vi "RockPaperScissors.vi"() -> ()   [LabVIEW 2021]
uses:
  <vilib>/numeric/Random Number (Range) DBL.vi
  <vilib>/Instr/_visa.llb/VISA Configure Serial Port (Instr).vi
panel:
  in  "Train":bool
  out "Output Selection 2":i32
  out "Output Selection 1":i32
  in  "Tab Control":enum32{"Play"}(tab)
  in  "Ready to Play":bool
  in  "User":picture
  in  "Computer":picture
  in  "Ring":u16(ring) items=["Scissors", "Paper", "Rock"]
  in  "Done":bool
  in  "VISA resource name":refnum<visa-resource-name>
  # "READY TO PLAY"
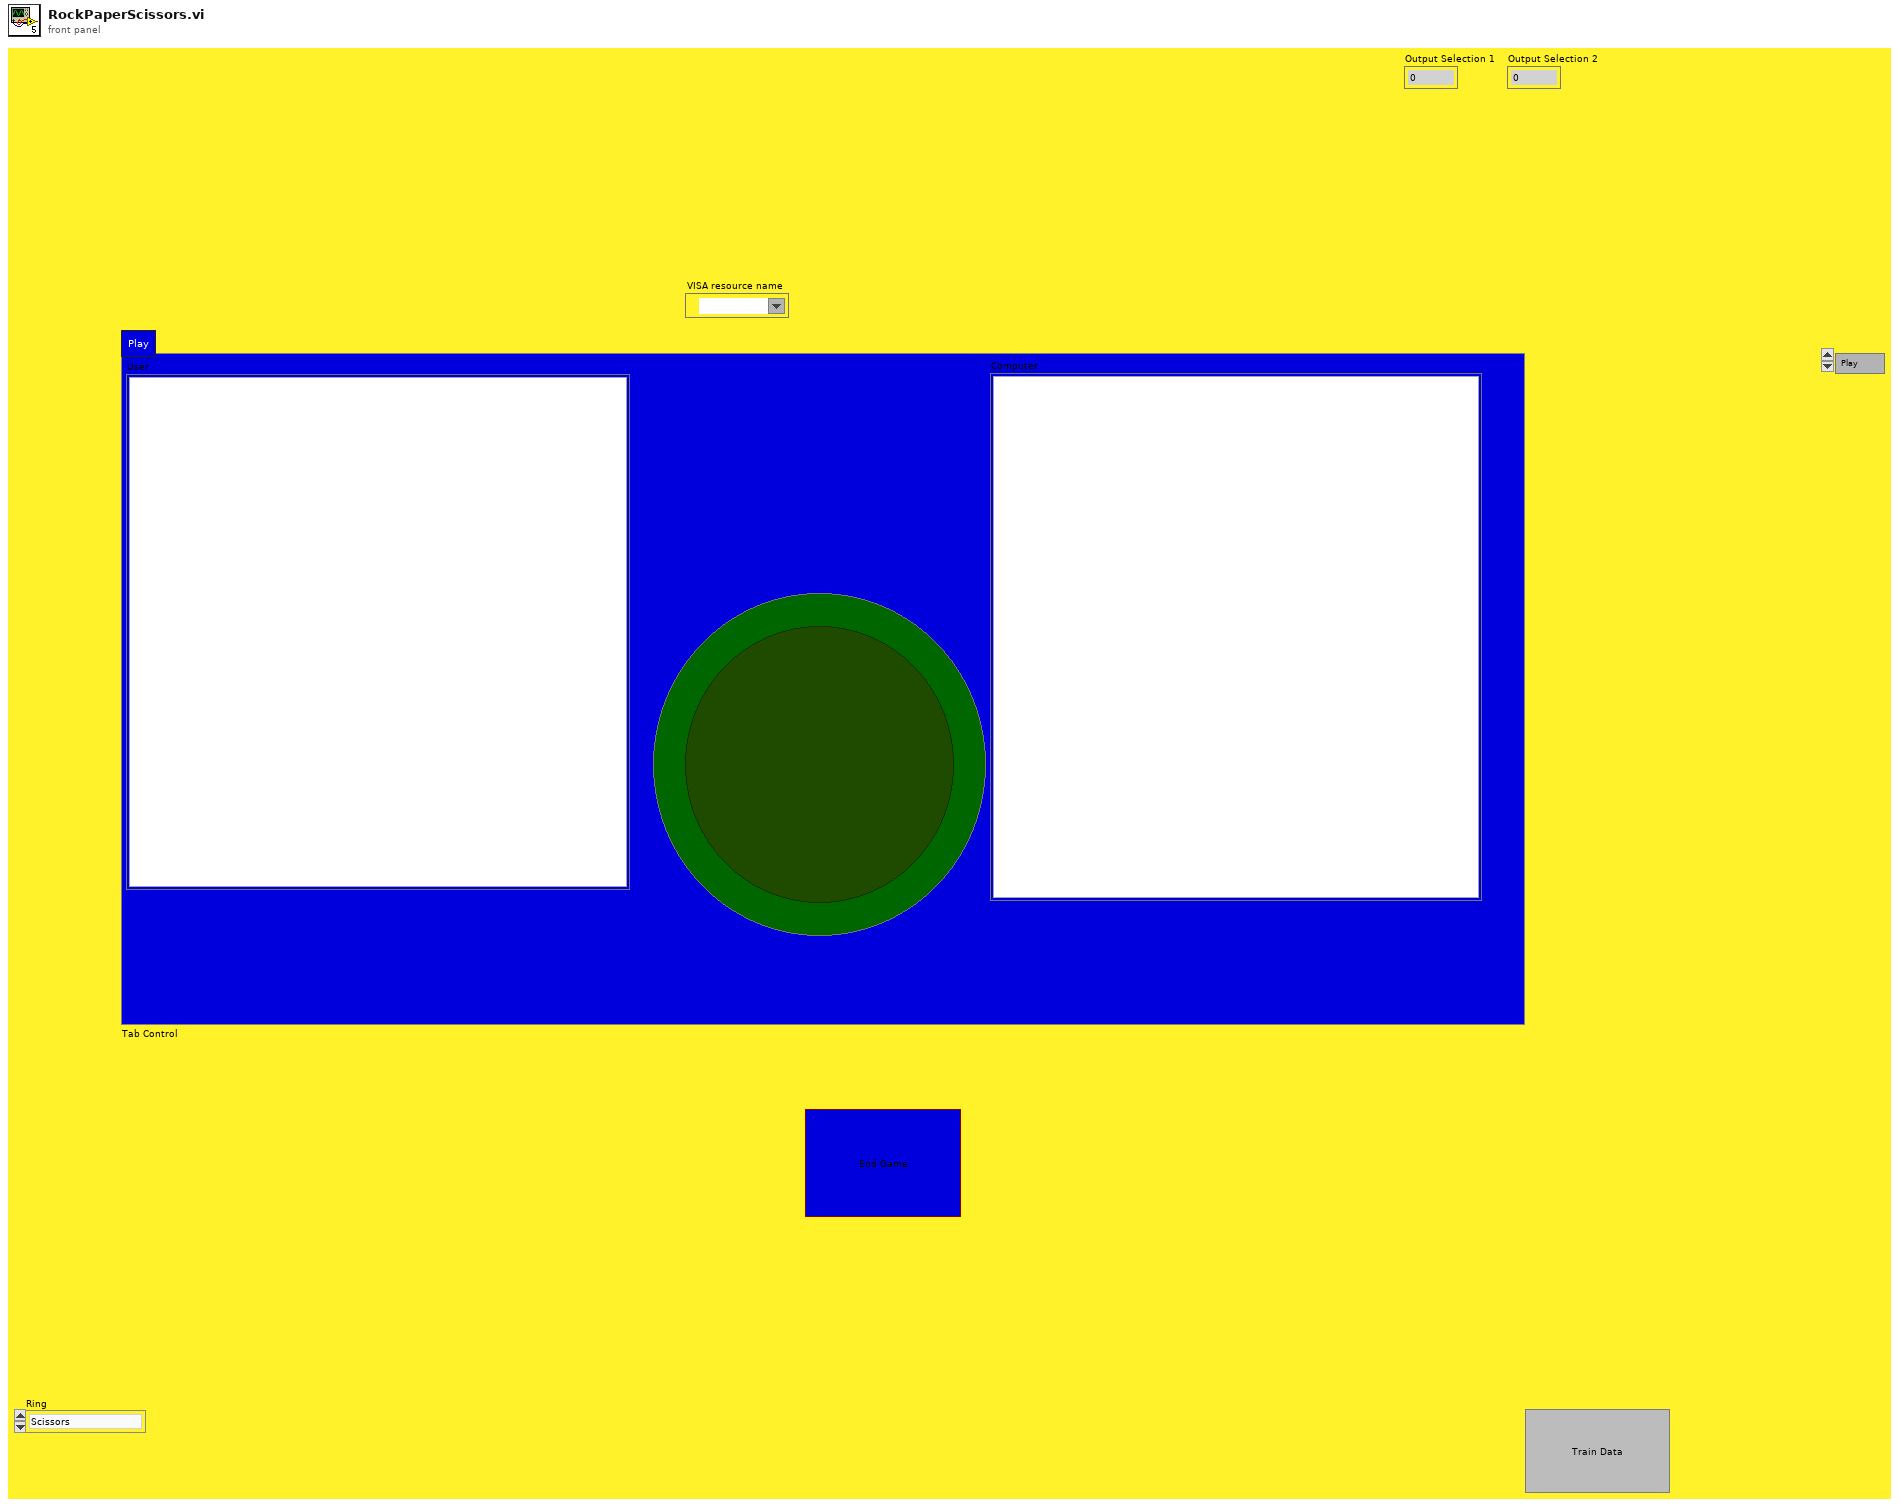
[diagram p1: front panel]
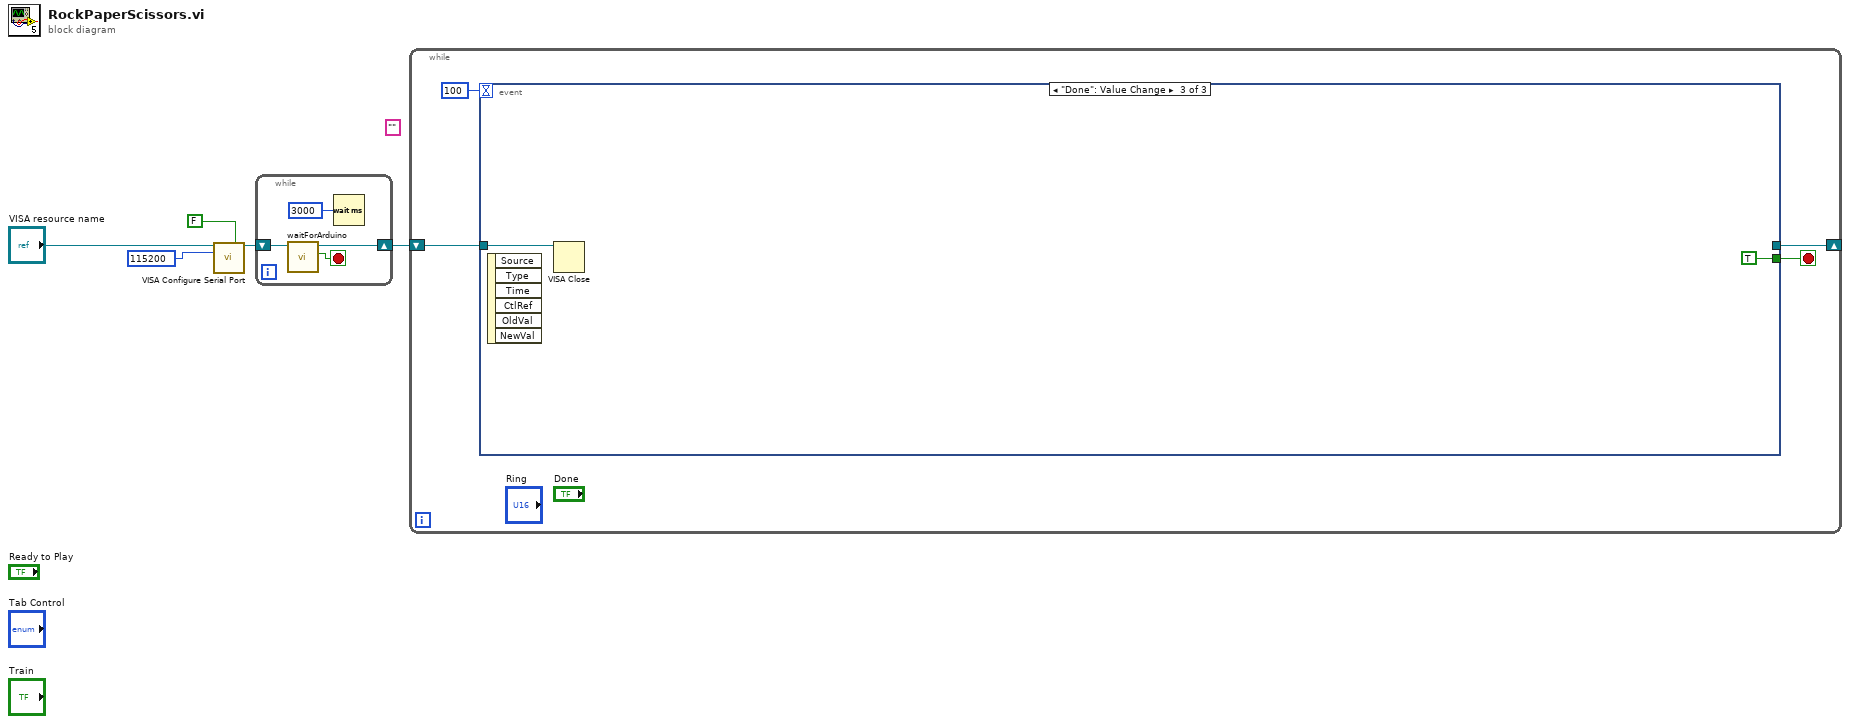
[diagram p0: block diagram]
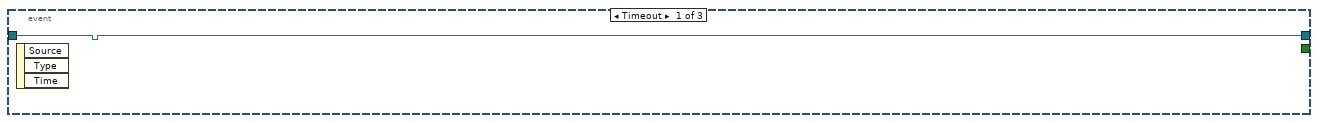
[diagram p2: hidden frame]
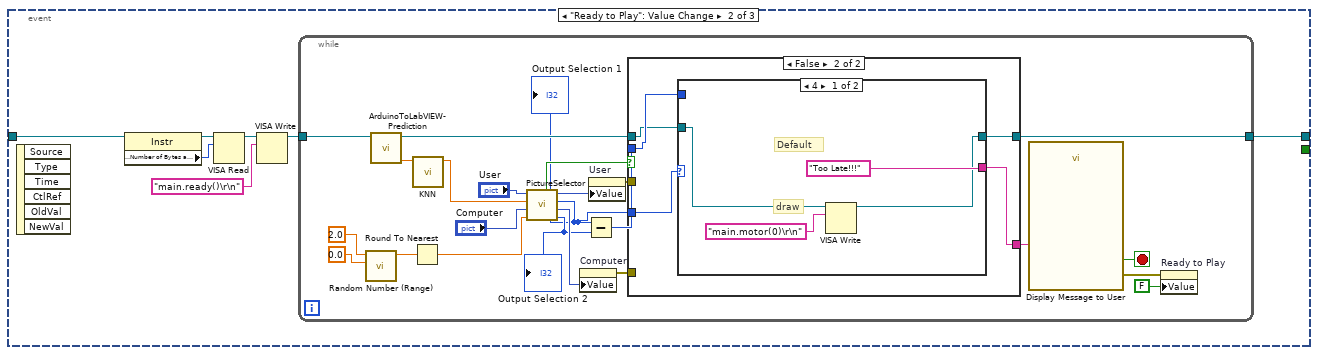
[diagram p3: hidden frame]
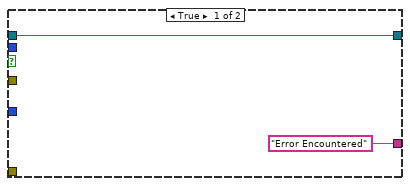
[diagram p4: hidden frame]
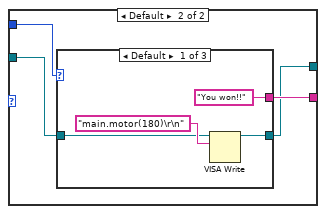
[diagram p5: hidden frame]
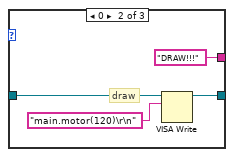
[diagram p6: hidden frame]
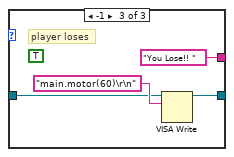
[diagram p7: hidden frame]
diagram:
  (unwired) ""
  n1 = call-poly "VISA Configure Serial Port"("VISA resource name"="VISA resource name", "Enable Termination\nChar (T)"=FALSE ("Enable Termination\nChar (T)"), "baud rate (9600)"=u32 115200) -> ("VISA resource name out"=w2:refnum<visa-resource-name>)  [unwired: 11 in, 1 out]
  n2 = while {
    shift-right: [w8] -> w1
    shift-left: w2 -> [w9]
    stop <- w7 stop-if-true
    n3 = call "waitForArduino.vi"("VISA Refnum in"=w9) -> ("Boolean"=w7:bool, "VISA Refnum out"=w8:refnum<visa-resource-name>)  [unwired: 9 in]
    n4 = Wait (ms)(milliseconds to wait=u32 3000) -> ()  [unwired: 1 out]
  }
  n5 = while {
    shift-right: [w11] -> _
    shift-left: w1 -> [w13]
    stop <- w12 stop-if-true
    n6 = event shown="[2] \"Done\": Value Change" {
      selector: _ -> [_ _ _]
      dyn-events: _ -> [_ _ _]
      timeout: 100 -> [_ _ _]
      tunnel: w13 -> [w14 w18 w72]
      tunnel: [_ _ TRUE] -> w12
      tunnel: [w14 w19 _] -> w11
      event Timeout {
        n7 = event-data() -> ()  [unwired: 1 in, 3 out]
      }
      event "Ready to Play": Value Change {
        n8 = event-data() -> ()  [unwired: 1 in, 6 out]
        n9 = property class="Instr"(reference=w18) -> (reference out=w17:refnum<visa-resource-name>, "Serial Settings:Number of Bytes at Serial Port"=w15:u32)  [unwired: 1 in, 1 out]
        n10 = VISA Read(VISA resource name=w17, byte count=w15) -> (VISA resource name out=w16:refnum<visa-resource-name>)  [unwired: 1 in, 3 out]
        n11 = VISA Write(VISA resource name=w16, write buffer="main.ready()\r\n") -> (VISA resource name out=w20:refnum<visa-resource-name>)  [unwired: 1 in, 2 out]
        n12 = while {
          tunnel: w20 -> [w33]
          tunnel: [w23] -> w19
          stop <- w37 stop-if-true
          n13 = call-poly <vilib>:"Random Number (Range).vi"("lower bound (0)"=0.0, "upper bound (100)"=2.0) -> ("number"=w41:dbl)  [unwired: 9 in]
          n14 = call "ArduinoToLabVIEW- Prediction.vi"("reference"=w33) -> ("SD"=w26:dbl, "VISA resource name out"=w24:refnum<visa-resource-name>)  [unwired: 9 in]
          n15 = Round To Nearest(number=w41) -> (nearest integer value=w32:dbl)
          n16 = call "KNN.vi"("SD from Arduino"=w26) -> ("element"=w25:dbl)  [unwired: 10 in]
          n17 = call "PictureSelector.vi"("Input Selection 2"=w32, "Input Picture 2"="Computer", "Input Selection 1"=w25, "Input Picture 1"="User") -> ("Output Selection 2"=w30:i32, "Output picture 2"=w31:picture, "Output Selection 1"=w22:i32, "Output picture"=w39:picture, "Error"=w36:bool)  [unwired: 3 in]
          "Output Selection 1" <- w22
          "Output Selection 2" <- w30
          n18 = property on="Computer" class="Pict"("Value"=w31) -> (error out=w27:errorcluster)  [unwired: 2 in, 1 out]
          n19 = Subtract(x=w22, y=w30) -> (x-y=w42:i32)
          n20 = property on="User" class="Pict"("Value"=w39) -> (error out=w28:errorcluster)  [unwired: 2 in, 1 out]
          n21 = case shown="False" w36 {
            tunnel: w42 -> [_ w51]
            tunnel: ["Error Encountered" ("Message") w50] -> w38
            tunnel: w28 -> [_ _]
            tunnel: w27 -> [_ _]
            tunnel: [w45 w49] -> w23
            tunnel: w24 -> [w45 w48]
            tunnel: w22 -> [_ w47]
            frame True {
            }
            frame False {
              n22 = case shown="4" w47 {
                tunnel: w51 -> [_ w59]
                tunnel: ["Too Late!!!" ("Message") w58] -> w50
                tunnel: [w53 w57] -> w49
                tunnel: w48 -> [w52 w56]
                frame 4 {
                  # "draw"
                  # "Default"
                  n23 = VISA Write(VISA resource name=w52, write buffer="main.motor(0)\r\n") -> (VISA resource name out=w53:refnum<visa-resource-name>)  [unwired: 1 in, 2 out]
                }
                frame Default {
                  n24 = case shown="Default" w59 {
                    tunnel: ["You won!!" ("Message") "DRAW!!!" ("Message") "You Lose!! " ("Message")] -> w58
                    tunnel: [w60 w65 w68] -> w57
                    tunnel: w56 -> [w61 w64 w69]
                    frame Default {
                      n25 = VISA Write(VISA resource name=w61, write buffer="main.motor(180)\r\n") -> (VISA resource name out=w60:refnum<visa-resource-name>)  [unwired: 1 in, 2 out]
                    }
                    frame 0 {
                      # "draw"
                      n26 = VISA Write(VISA resource name=w64, write buffer="main.motor(120)\r\n") -> (VISA resource name out=w65:refnum<visa-resource-name>)  [unwired: 1 in, 2 out]
                    }
                    frame -1 {
                      (unwired) TRUE
                      # "player loses"
                      n27 = VISA Write(VISA resource name=w69, write buffer="main.motor(60)\r\n") -> (VISA resource name out=w68:refnum<visa-resource-name>)  [unwired: 1 in, 2 out]
                    }
                  }
                }
              }
            }
          }
          n28 = call "Display Message to User"("Message"=w38) -> ("error out"=w34:errorcluster, "OK"=w37:bool)  [unwired: 9 in]
          n29 = property on="Ready to Play" class="Bool (strict)"(error in=w34, "Value"=FALSE ("Ready to Play")) -> ()  [unwired: 1 in, 2 out]
        }
      }
      event "Done": Value Change {
        n30 = event-data() -> ()  [unwired: 1 in, 6 out]
        n31 = VISA Close(VISA resource name=w72) -> ()  [unwired: 1 in, 1 out]
      }
    }
  }
